vi "Dashboard Main.vi"() -> ()   [LabVIEW 2013]
uses:
  <vilib>/event_ctls.llb/eventvkey.ctl
  <vilib>/Rock Robotics/WPI/Dashboard/WPI_DashboardLogging Global.vi
  <vilib>/Utility/config.llb/Write Key (String).vi
  <vilib>/Utility/config.llb/Write Key (I32).vi
  <vilib>/Utility/config.llb/NI_LVConfig.lvlib
  <vilib>/vision/NI_Vision_Development_Module.lvlib
panel:
  out "Image Message":string="Timeout in Camera Communications"
  in  "Rec Mode":enum32{"Stop", "Record", "Playback"}(radio)
  in  "Dashboard Tab":T1(tab)=enum."Auto"
  out "SHOOT":bool
  in  "Camera Settings":T2={"Frame Rate"=7, "Compression"=0, "Size"=1} {"Frame Rate" scale=1.0..30.0; "Size" items=["640x480", "320x240", "160x120"]}
  out "MotorSliders R":cluster{"MotorSlide1":dbl, "MotorSlide2":dbl} {"MotorSlide2" scale=-1.0..1.0 scale format="%#_2e"; "MotorSlide1" scale=-1.0..1.0 scale format="%#_2e"}
  out "MotorChart R":cluster{"Numeric":dbl, "Numeric":dbl}(graph)
  out "MotorSliders L":T3 {"MotorSlide4 2" scale=0.0..14.0 scale format="%#_2e"; "MotorSlide2" scale=-1.0..1.0 scale format="%#_2e"; "MotorSlide1" scale=-1.0..1.0 scale format="%#_2e"}
  out "MotorChart L":T4(graph)
  out "JS1 Z":dbl(slide) scale=-1.0..1.0 scale format="%#_2e"
  out "Joystick 1":cluster{"X":dbl, "Y":dbl}[](graph)
  out "JS Buttons 1":T5
  out "JS2 Z":dbl(slide) scale=-1.0..1.0 scale format="%#_2e"
  out "Joystick 2":cluster{"X":dbl, "Y":dbl}[](graph)
  out "JS Buttons 2":T5
  out "Mode":T6(ring)=enum.""
  in  "DB Camera Config":bool
  out "fps":dbl format="%#.1g"
  out "Mbps":dbl format="%#.1g"
  out "Mbps 2":bool
  out "LED 1":bool
  out "Camera IP Address":string="0.0.0.11"
  in  "Bunches of Variables":T7={"Parameter 1"=1.0596, "Parameter 2"=-19.179, "Camera view angle"=33.7} {"Camera view angle" format="%#_13g"}
  out "Number of Particles":i32=1
  in  "Color Mode":u16(ring)=1 items=["RGB", "HSL", "HSV", "HSI"]
  out "Distance (in)":dbl
  in  "Filter ON":bool
  in  "Green or Saturation":cluster{i32, i32}(slide)={44, 255} scale=0.0..255.0
  in  "Blue or Luminance":cluster{i32, i32}(slide)={147, 255} scale=0.0..255.0
  in  "Red or Hue":cluster{i32, i32}(slide)={89, 148} scale=0.0..255.0
  in  "Combo Box":string(combo)="Custom"
  out "Tallest Area":dbl
  out "Widest Area":dbl
  out "Hot":bool
  in  "Test Slider":dbl(slide) scale=0.0..100.0 scale format="%#_3g"
  in  "On/Off":bool caption="Solenoid"
  in  "Test Name":u16(ring) items=["Select the test to run...", "Example Test", "-------------------------------", "List of tests is built in robot code.", "Replace with your own automated tests."]
  in  "Test Tree":string(tree)
  in  "Motor":cluster{"Value":dbl, "Enable":bool} {"Value" scale=-1.0..1.0 scale format="%#_3g"}
  out "Progress":T8 {"Test Progress" scale=0.0..100.0}
  in  "Rev/Fwd":cluster{"Forward":bool, "Reverse":bool}
  in  "Test Ring":u16(ring) items=["Auto", "Fixed indoor", "Fixed outdoor 1", "Fixed outdoor 2", "Fixed fluorescent 1", "Fixed fluorescent 2", "Hold current"]
  in  "Listbox":i32(listbox)
  out "Tree":string(tree)
  out "Camera Image":T9(plugin-control)
  # "Left"
  # "Front"
  # "Right"
  # "Battery"
  # "Customize by placing controls and indicators here and name to\nmatch Dashboard Variables on robot."
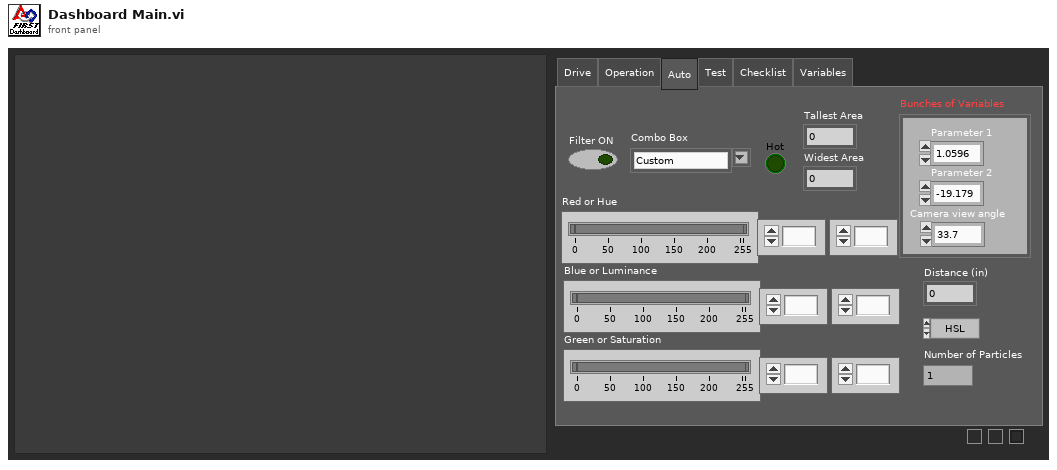
[diagram p1: front panel]
types:
  T1 = enum32{"Drive", "Operation", "Auto", "Test", "Checklist", "Variables"}
  T2 = cluster{"Frame Rate":i32, "Compression":i32, "Size":u16}
  T3 = cluster{"MotorSlide1":dbl, "MotorSlide2":dbl, "MotorSlide4 2":dbl}
  T4 = cluster{"Numeric":dbl, "Numeric":dbl, "Battery":sgl}
  T5 = cluster{bool, bool, bool, bool, bool, bool, bool, bool, bool, bool, bool, bool}
  T6 = enum8{"Tele-Op Disabled", "Tele-Op Enabled", "Auto Disabled", "Auto Enabled", "Test Disabled", "Test Enabled", ""}
  T7 = cluster{"Parameter 1":dbl, "Parameter 2":dbl, "Camera view angle":dbl}
  T8 = cluster{"Test Progress":u8, "Test Progress Text":string}
  T9 = typedef "IMAQ Image.ctl" = refnum<image>
  T10 = typedef "Image Type" = u32
  T11 = cluster{"Digital Inputs":bool[], "Digital Outputs":bool[]}
  T12 = cluster{"Competition mode":bool, "Robot Link":bool, "Autonomous":bool, "Enabled":bool, "E-Stop":bool, "Simulated":bool, "TestMode":bool, "Docked Window":bool}
  T13 = cluster{"Boolean Array[0]":bool, "Boolean Array[1]":bool, "Boolean Array[2]":bool, "Boolean Array[3]":bool, "Boolean Array[4]":bool, "Boolean Array[5]":bool, "Boolean Array[6]":bool, "Boolean Array[7]":bool, "Boolean Array[8]":bool, "Boolean Array[9]":bool, "Boolean Array[10]":bool, "Boolean Array[11]":bool}
  T14 = typedef "NI_LVConfig.lvlib/Config Data RefNum.ctl" = refnum<k1>
  T15 = typedef "eventvkey.ctl" = enum16{"ASCII", "Enter", "Return", "Shift", "Ctrl", "Alt", "Cmd", "Opt", "Caps", "NumLock", "Clear", "Break", "Up", "Down", "Left", "Right", "Insert", "Delete", "Home", "End", "PageUp", "PageDown", "Escape", "Help", "Pause", "ScrollLock", "F1", "F2", "F3", "F4", "F5", "F6", "F7", "F8", "F9", "F10", "F11", "F12", "F13", "F14", "F15", "F16", "F17", "F18", "F19", "F20", "F21", "F22", "F23", "F24", "Play", "VolumeUp", "VolumeDown", "Mute", "Two Byte Char"}
  T16 = cluster{"Image Size":bool, "Image Type":bool, "Pixel Value":bool, "ROI Information":bool, "Zoom Factor":bool}
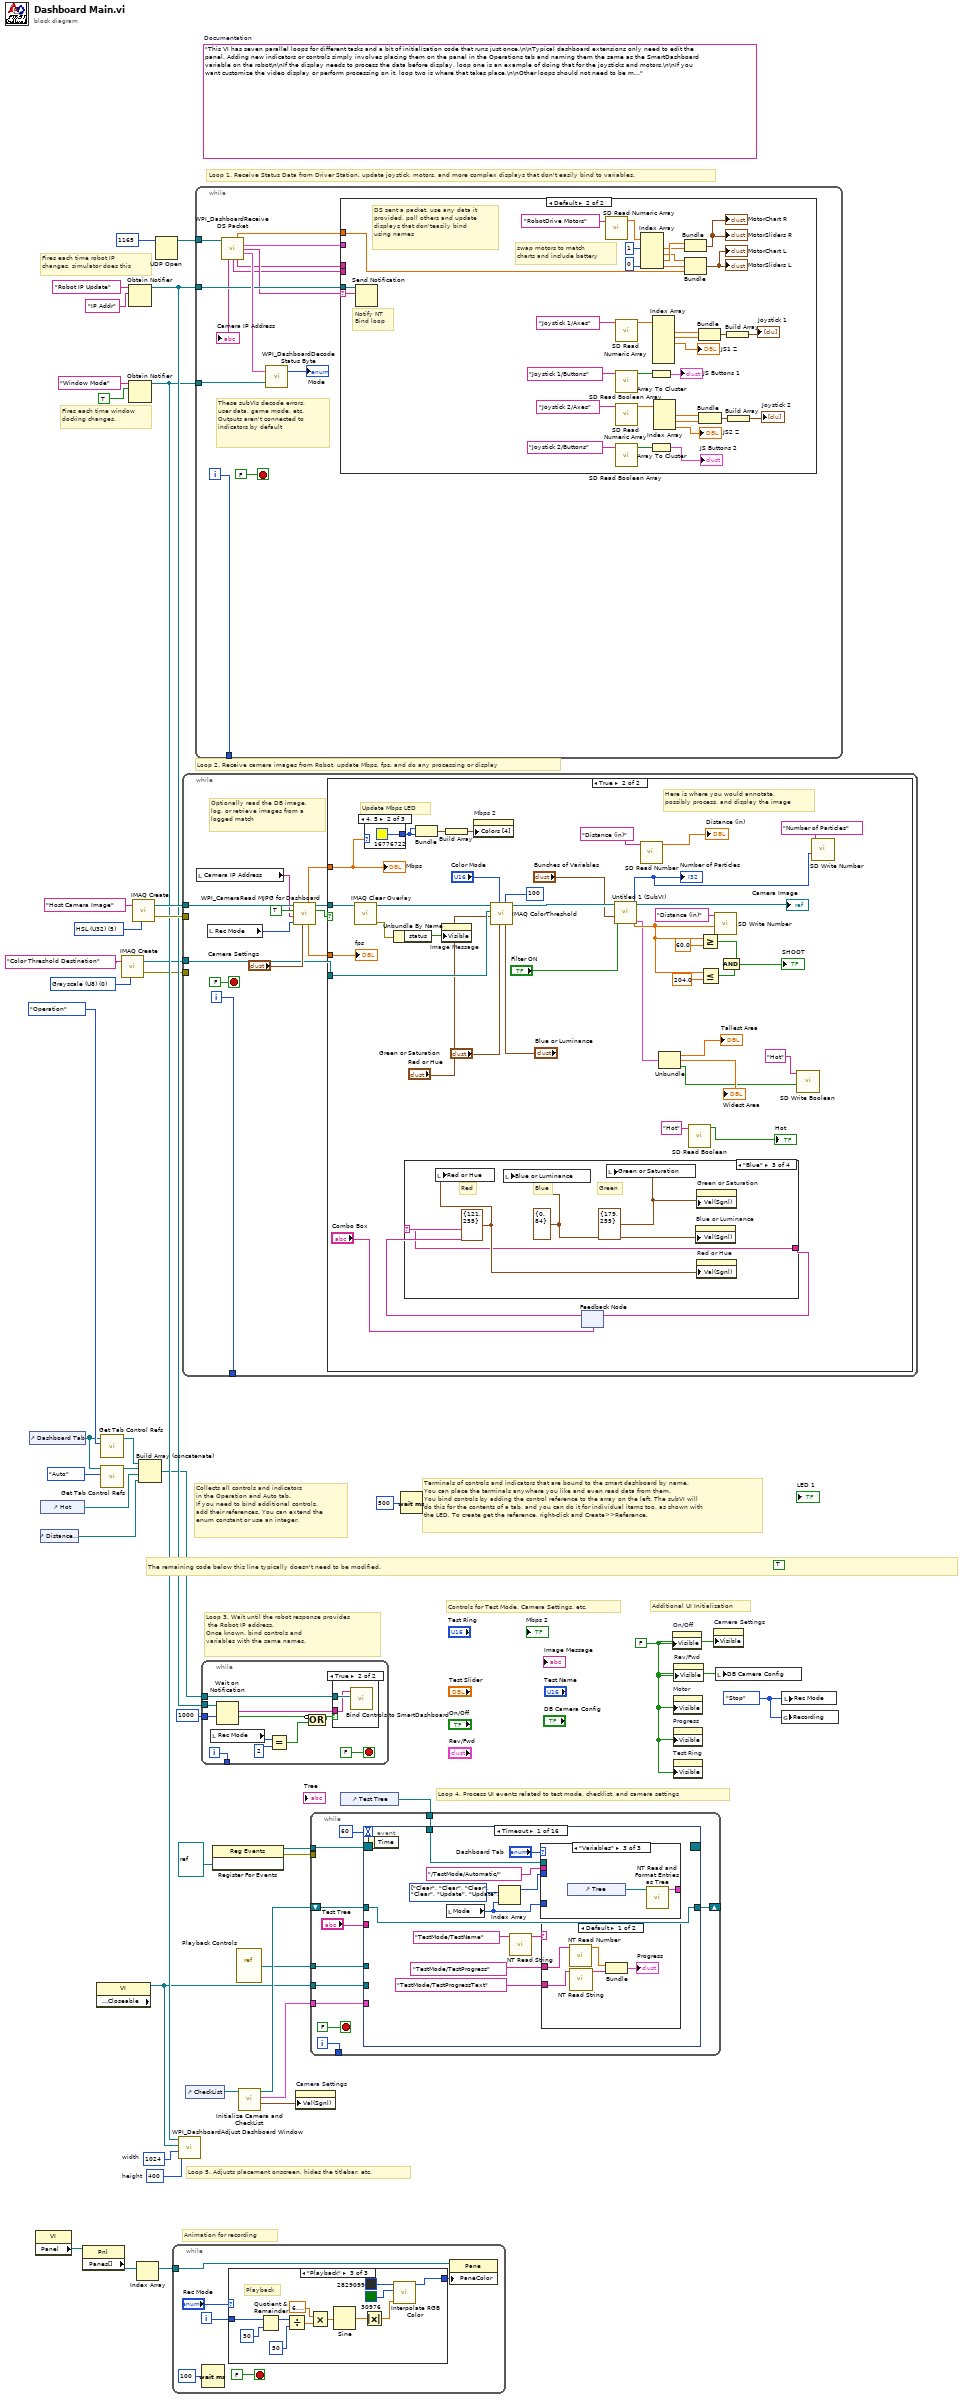
[diagram p0: block diagram]
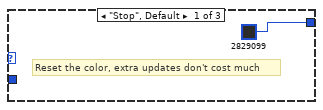
[diagram p2: hidden frame]
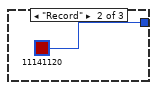
[diagram p3: hidden frame]
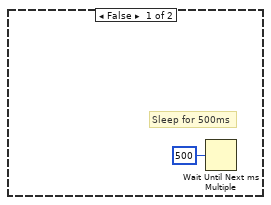
[diagram p5: hidden frame]
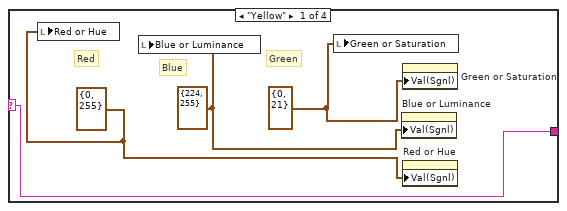
[diagram p6: hidden frame]
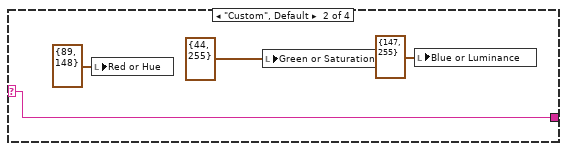
[diagram p7: hidden frame]
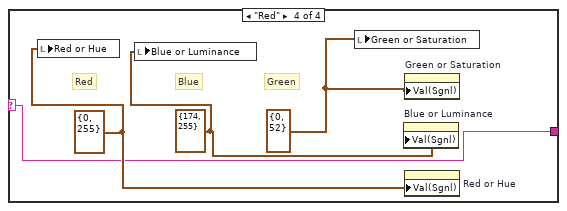
[diagram p8: hidden frame]
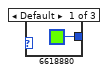
[diagram p9: hidden frame]
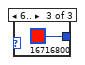
[diagram p10: hidden frame]
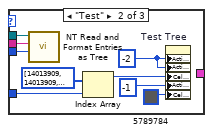
[diagram p12: hidden frame]
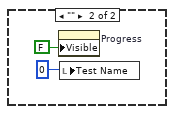
[diagram p13: hidden frame]
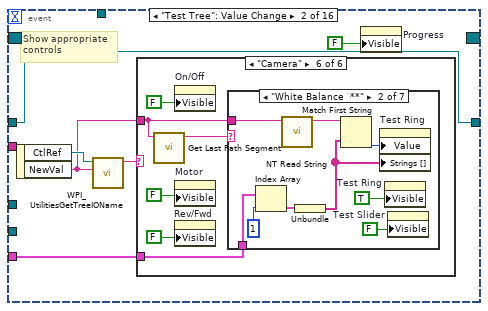
[diagram p14: hidden frame]
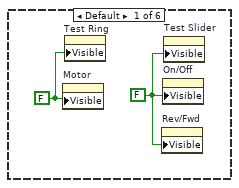
[diagram p15: hidden frame]
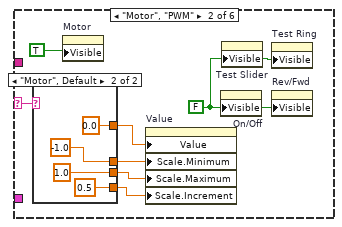
[diagram p16: hidden frame]
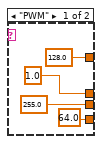
[diagram p17: hidden frame]
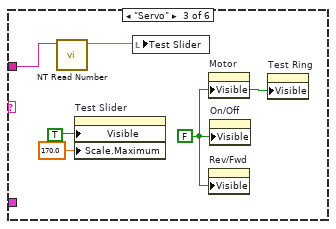
[diagram p18: hidden frame]
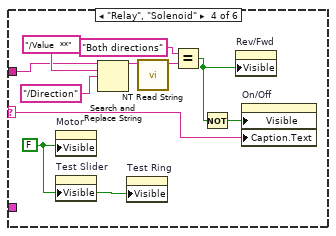
[diagram p19: hidden frame]
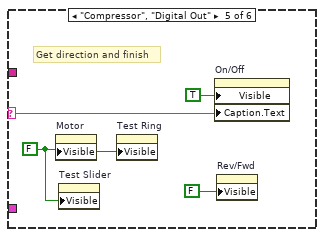
[diagram p20: hidden frame]
diagram:
  (unwired) TRUE
  w6 = T10 0 items=["Grayscale (U8)", "Grayscale (I16)", "Grayscale (SGL)", "Complex (CSG)", "RGB (U32)", "HSL (U32)", "RGB (U64)", "Grayscale (U16)"] ("Image Type")
  w14 = enum32{"Stop", "Record", "Playback"}."Stop" ("Rec Mode")
  w17 = 400  # height
  w18 = 1024  # width
  w31 = FALSE ("Visible")
  (unwired) "This VI has seven parallel loops for different tasks and a bit of initialization code that runs just once.\n\nTypical dashboard extensions only need to edit the panel. Adding new indicators or controls simply involves placing them on the panel in the Operations tab and naming them the same as the SmartDashboard variable on the robot\n\nIf the display needs to process the data before display, loop one is an example of doing that for the joysticks and motors.\n\nIf you want customize the video display or perform processing on it, loop two is where that takes place.\n\nOther loops should not need to be modified. They are pretty standard, and document the task they perform."  # Documentation
  w41 = T10 5 items=["Grayscale (U8)", "Grayscale (I16)", "Grayscale (SGL)", "Complex (CSG)", "RGB (U32)", "HSL (U32)", "RGB (U64)"] ("Image Type")
  # "Controls for Test Mode, Camera Settings, etc."
  # "Additional UI Initialization"
  # "Animation for recording"
  # "Fires each time robot IP\nchanges, simulator does this"
  # "Fires each time window\ndocking changes."
  # "Collects all controls and indicators\nin the Operation and Auto tab.\nIf you need to bind additional controls,\nadd their references. You can extend the\nenum constant or use an integer."
  # "The remaining code below this line typically doesn't need to be modified."
  # "Loop 4. Process UI events related to test mode, checklist, and camera settings"
  # "Terminals of controls and indicators that are bound to the smart dashboard by name.\nYou can place the terminals anywhere you like and even read data from them.\nYou bind controls by adding the control reference to the array on the left. The subVI will\ndo this for the contents of a tab, and you can do it for individual items too, as shown with\nthe LED. To create get the reference, right-click and Create>>Reference."
  # "Loop 3. Wait until the robot response provides\n the Robot IP address.\nOnce known, bind controls and\nvariables with the same names."
  # "Loop 5. Adjusts placement onscreen, hides the titlebar, etc."
  # "Loop 1. Receive Status Data from Driver Station, update joystick, motors, and more complex displays that don't easily bind to variables."
  # "Loop 2. Receive camera images from Robot, update Mbps, fps, and do any processing or display"
  n1 = control-ref of="Dashboard Tab"() -> (w12:refnum<vi>)
  n2 = property class="VI"() -> ("Panel"=w25:refnum<vi>)  [unwired: 2 in, 2 out]
  n3 = control-ref of="Hot"() -> (w7:refnum<vi>)
  n4 = control-ref of="Distance (in)"() -> (w2:refnum<vi>)
  n5 = property class="Pnl"(reference=w25) -> ("Panes[]"=w26:refnum<vi>[])  [unwired: 1 in, 2 out]
  n6 = property class="VI" props=["Front Panel.Closeable"]() -> (reference out=w13:refnum<vi>)  [unwired: 2 in, 2 out]
  n7 = call <vilib>:"Get Tab Control Refs.vi"("Page Index"=T1."Operation" ("Dashboard Tab"), "TabControl in"=w12) -> ("ControlsOnPage"=w10:refnum<vi>[])  [unwired: 9 in]
  n8 = call <vilib>:"Get Tab Control Refs.vi"("Page Index"=T1."Auto" ("Dashboard Tab"), "TabControl in"=w12) -> ("ControlsOnPage"=w11:refnum<vi>[])  [unwired: 9 in]
  n9 = call "IMAQ Create"("Image Name"="Color Threshold Destination", "Image Type"=w6) -> ("New Image"=w5:T9, "error out"=w4:errorcluster)  [unwired: 3 in]
  n10 = Obtain Notifier(name (unnamed)="Robot IP Update", notification data type="IP Addr" ("name (unnamed)")) -> (notifier out=w35:refnum<notifier>)  [unwired: 2 in, 2 out]
  n11 = Obtain Notifier(name (unnamed)="Window Mode", notification data type=TRUE) -> (notifier out=w16:refnum<notifier>)  [unwired: 2 in, 2 out]
  n12 = call "IMAQ Create"("Image Name"="Host Camera Image", "Image Type"=w41) -> ("New Image"=w39:T9, "error out"=w38:errorcluster)  [unwired: 2 in, 1 out]
  n13 = Index Array(array=w26) -> (element=w24:refnum<vi>)  [unwired: 1 in]
  n14 = Build Array (concatenate)(w10, w11, w7, w2) -> (w9:refnum<vi>[])
  n15 = UDP Open(11:u16 1165 ("port")) -> (port=w42:refnum<k16>)  [unwired: 2 in, 4 out]
  n16 = while {
    tunnel: w24 -> [w45]
    i -> [w48]
    stop <- FALSE stop-if-true
    n17 = Wait (ms)(milliseconds to wait=u32 100) -> ()  [unwired: 1 out]
    n18 = case shown="\"Playback\"" "Rec Mode" {
      tunnel: w48 -> [_ _ w63]
      tunnel: [u32 2829099 ("Base Color") u32 11141120 ("Target Color") w52] -> w44
      frame "Stop", Default {
        # "Reset the color, extra updates don't cost much"
      }
      frame "Record" {
      }
      frame "Playback" {
        # "Playback"
        n19 = Quotient & Remainder(x=w63, y=u32 50 ("milliseconds to wait")) -> (x-y*floor(x/y)=w59:u32)  [unwired: 1 out]
        n20 = Divide(x=w59, y=u32 50 ("milliseconds to wait")) -> (x/y=w56:dbl)
        n21 = Multiply(x=6.283185307179586, y=w56) -> (x*y=w61:dbl)
        n22 = Sine(x=w61) -> (sin(x)=w60:dbl)
        n23 = Absolute Value(x=w60) -> (abs(x)=w53:dbl)
        n24 = call "Interpolate RGB Color.vi"("Proportion"=w53, "Target Color"=u32 30976, "Base Color"=u32 2829099) -> ("Result Color"=w52:u32)  [unwired: 8 in]
      }
    }
    n25 = property class="Pane"(reference=w45, "PaneColor"=w44) -> ()  [unwired: 1 in, 2 out]
  }
  n26 = call <vilib>:"WPI_DashboardAdjust Dashboard Window.vi"("height"=w17, "width"=w18, "reference in"=w13, "Notifier in"=w16) -> ()  [unwired: 8 in]
  n27 = while {
    tunnel: w39 -> [w73]
    tunnel: w38 -> [_]
    tunnel: [w74] -> _
    tunnel: w5 -> [w66]
    tunnel: w4 -> [_]
    i -> [w74]
    stop <- FALSE stop-if-true
    # "Optionally read the DB image,\nlog, or retrieve images from a\nlogged match"
    n28 = local read "Camera IP Address"() -> (w64:string)
    n29 = local read "Rec Mode"() -> (w65:enum32{"Stop", "Record", "Playback"})
    n30 = call <vilib>:"WPI_CameraRead MJPG for Dashboard.vi"("Camera Settings"="Camera Settings", "Rec Mode"=w65, "Camera IP"=w64, "Enable"=TRUE, "Refnum in"=w73) -> ("Active"=w70:bool, "Refnum out"=w72:T9, "FPS"=w69:dbl, "Bandwidth (Mbps)"=w68:dbl)  [unwired: 3 in]
    n31 = case shown="True" w70 {
      tunnel: w72 -> [_ w111]
      tunnel: w68 -> [_ w110]
      tunnel: w69 -> [_ w109]
      tunnel: w66 -> [_ w106]
      frame False {
        # "Sleep for 500ms"
        n32 = Wait Until Next ms Multiple(millisecond multiple=u32 500) -> ()  [unwired: 1 out]
      }
      frame True {
        # "Here is where you would annotate,\npossibly process, and display the image"
        # "Update Mbps LED"
        n33 = call "IMAQ Clear Overlay"("Image"=w111) -> ("error out"=w115:errorcluster, "Image Out"=w105:T9)  [unwired: 2 in, 7 out]
        n34 = case shown="4, 5" w110 {
          tunnel: [u32 6618880 ("Color Box") u32 16776722 ("Color Box") u32 16716800 ("Color Box")] -> w112
          frame Default {
          }
          frame 4, 5 {
          }
          frame 6.. {
          }
        }
        n35 = Unbundle By Name(w115) -> ("status"=w116:bool)
        n36 = Bundle("Color Box"=w112, "Color Box"=w112) -> (w114:cluster{"Color Box":u32, "Color Box":u32})  [unwired: 1 out]
        n37 = property on="Image Message" class="Str"("Visible"=w116) -> ()  [unwired: 2 in, 2 out]
        n38 = Build Array(w114) -> (w113:cluster{"Color Box":u32, "Color Box":u32}[])
        n39 = property on="Mbps 2" class="Bool (strict)"("Colors [4]"=w113) -> ()  [unwired: 2 in, 2 out]
        n40 = call "IMAQ ColorThreshold"("Blue or Luma or Val or Inten Range"="Blue or Luminance", "Replace Value"=100, "Green or Sat Range"="Green or Saturation", "Color Mode"="Color Mode", "Red or Hue Range"="Red or Hue", "Image Dst"=w106, "Image Src"=w105) -> ("Image Dst Out"=w104:T9)  [unwired: 3 in, 1 out]
        n41 = feedback #1("Combo Box") -> (w84:string)
        n42 = case shown="\"Blue\"" w84 {
          selector: w84 -> [w117 w121 w125 w129]
          tunnel: [w117 w121 w125 w129] -> w85
          frame "Yellow" {
            w118 = cluster{"Lower value":i32, "Upper value":i32} {"Lower value"=0, "Upper value"=21} ("Red or Hue Range")
            w119 = cluster{"Lower value":i32, "Upper value":i32} {"Lower value"=224, "Upper value"=255} ("Red or Hue Range")
            w120 = cluster{"Lower value":i32, "Upper value":i32} {"Lower value"=0, "Upper value"=255} ("Red or Hue Range")
            # "Green"
            # "Blue"
            # "Red"
            n43 = local write "Red or Hue"(w120) -> ()
            n44 = local write "Blue or Luminance"(w119) -> ()
            n45 = local write "Green or Saturation"(w118) -> ()
            n46 = property on="Blue or Luminance" class="Slide (strict)"("Val(Sgnl)"=w119) -> ()  [unwired: 2 in, 2 out]
            n47 = property on="Green or Saturation" class="Slide (strict)"("Val(Sgnl)"=w118) -> ()  [unwired: 2 in, 2 out]
            n48 = property on="Red or Hue" class="Slide (strict)"("Val(Sgnl)"=w120) -> ()  [unwired: 2 in, 2 out]
          }
          frame "Custom", Default {
            n49 = local write "Red or Hue"(cluster{i32, i32} {89, 148} ("Red or Hue")) -> ()
            n50 = local write "Green or Saturation"(cluster{i32, i32} {44, 255} ("Green or Saturation")) -> ()
            n51 = local write "Blue or Luminance"(cluster{i32, i32} {147, 255} ("Blue or Luminance")) -> ()
          }
          frame "Blue" {
            w127 = cluster{"Lower value":i32, "Upper value":i32} {"Lower value"=179, "Upper value"=255} ("Red or Hue Range")
            w128 = cluster{"Lower value":i32, "Upper value":i32} {"Lower value"=0, "Upper value"=84} ("Red or Hue Range")
            w126 = cluster{"Lower value":i32, "Upper value":i32} {"Lower value"=121, "Upper value"=255} ("Red or Hue Range")
            # "Green"
            # "Blue"
            # "Red"
            n52 = local write "Red or Hue"(w126) -> ()
            n53 = local write "Blue or Luminance"(w128) -> ()
            n54 = local write "Green or Saturation"(w127) -> ()
            n55 = property on="Blue or Luminance" class="Slide (strict)"("Val(Sgnl)"=w128) -> ()  [unwired: 2 in, 2 out]
            n56 = property on="Green or Saturation" class="Slide (strict)"("Val(Sgnl)"=w127) -> ()  [unwired: 2 in, 2 out]
            n57 = property on="Red or Hue" class="Slide (strict)"("Val(Sgnl)"=w126) -> ()  [unwired: 2 in, 2 out]
          }
          frame "Red" {
            w131 = cluster{"Lower value":i32, "Upper value":i32} {"Lower value"=0, "Upper value"=52} ("Red or Hue Range")
            w132 = cluster{"Lower value":i32, "Upper value":i32} {"Lower value"=174, "Upper value"=255} ("Red or Hue Range")
            w130 = cluster{"Lower value":i32, "Upper value":i32} {"Lower value"=0, "Upper value"=255} ("Red or Hue Range")
            # "Green"
            # "Blue"
            # "Red"
            n58 = local write "Red or Hue"(w130) -> ()
            n59 = local write "Blue or Luminance"(w132) -> ()
            n60 = local write "Green or Saturation"(w131) -> ()
            n61 = property on="Blue or Luminance" class="Slide (strict)"("Val(Sgnl)"=w132) -> ()  [unwired: 2 in, 2 out]
            n62 = property on="Green or Saturation" class="Slide (strict)"("Val(Sgnl)"=w131) -> ()  [unwired: 2 in, 2 out]
            n63 = property on="Red or Hue" class="Slide (strict)"("Val(Sgnl)"=w130) -> ()  [unwired: 2 in, 2 out]
          }
        }
        n64 = feedback-in #1(w85) -> ()
        n65 = call "Untitled 1 (SubVI).vi"("Filter ON"="Filter ON", "Cluster"="Bunches of Variables", "Image Dst Out"=w104, "Refnum in"=w105) -> ("output cluster"=w88:cluster{dbl, dbl, bool}, "Distance (in)"=w94:dbl, "Number of Particles"=w77:i32, "Refnum out"=→"Camera Image":T9)  [unwired: 4 in]
        "Number of Particles" <- w77
        n66 = call <vilib>:"SD Read Number.vi"("Name"="Distance (in)") -> ("Numeric"=→"Distance (in)":dbl)  [unwired: 8 in, 2 out]
        n67 = Unbundle(w88) -> (→"Tallest Area":dbl, →"Widest Area":dbl, w82:bool)
        n68 = call <vilib>:"SD Read Boolean.vi"("Name"="Hot") -> ("Boolean"=→"Hot":bool)  [unwired: 8 in, 2 out]
        n69 = Greater Or Equal?(x=w94, y=60.0) -> (x >= y?=w102:bool)
        n70 = Less Or Equal?(x=w94, y=204.0) -> (x <= y?=w100:bool)
        n71 = call <vilib>:"SD Write Number.vi"("Numeric"=w94, "Name"="Distance (in)") -> ()  [unwired: 8 in, 2 out]
        n72 = And(x=w102, y=w100) -> (x .and. y?=→"SHOOT":bool)
        n73 = call <vilib>:"SD Write Boolean.vi"("Boolean"=w82, "Name"="Hot") -> ()  [unwired: 8 in, 2 out]
        n74 = call <vilib>:"SD Write Number.vi"("Numeric"=w77, "Name"="Number of Particles") -> ()  [unwired: 8 in, 2 out]
        "Mbps" <- w110
        "fps" <- w109
      }
    }
  }
  n75 = control-ref of="CheckList"() -> (w15:refnum<vi>)
  n76 = while {
    tunnel: w42 -> [w146]
    tunnel: w35 -> [w142]
    tunnel: w16 -> [w145]
    tunnel: [w143] -> _
    i -> [w143]
    stop <- FALSE stop-if-true
    # "These subVIs decode errors, user data, game mode, etc.\nOutputs aren't connected to indicators by default"
    n77 = call <vilib>:"WPI_DashboardReceive DS Packet.vi"("Recv Socket"=w146) -> ("Battery"=w137:sgl, "Driver Station"=w138:T11, "Robot IP Address"=w141:string, "Status"=w147:T12, "Camera IP Address"=→"Camera IP Address":string, "Low Priority User Data"=w140:string, "High Priority User Data"=w139:string)  [unwired: 1 in, 7 out]
    n78 = call <vilib>:"WPI_DashboardDecode Status Byte.vi"("Window Mode Notifier"=w145, "Status"=w147) -> ("Mode"=→"Mode":T6)  [unwired: 1 out]
    n79 = case shown="Default" w141 {
      selector: w141 -> [_ w159]
      tunnel: w142 -> [_ w160]
      tunnel: w140 -> [_ _]
      tunnel: w139 -> [_ _]
      tunnel: w138 -> [_ _]
      tunnel: w137 -> [_ w158]
      frame "0.0.0.0" {
        # "DS not sending packets, or no robot exists yet.\nDon't poll the variables"
      }
      frame Default {
        # "Notify NT\nBind loop"
        # "DS sent a packet. use any data it\nprovided, poll others and update\ndisplays that don'teasily bind\nusing names"
        # "swap motors to match\ncharts and include battery"
        n80 = Send Notification(notification=w159, notifier=w160) -> ()  [unwired: 1 in, 2 out]
        n81 = call <vilib>:"SD Read Numeric Array.vi"("Name"="RobotDrive Motors") -> ("Numeric Array"=w157:dbl[])  [unwired: 8 in, 2 out]
        n82 = call <vilib>:"SD Read Numeric Array.vi"("Name"="Joystick 1/Axes") -> ("Numeric Array"=w176:dbl[])  [unwired: 8 in, 2 out]
        n83 = call <vilib>:"SD Read Boolean Array.vi"("Name"="Joystick 1/Buttons") -> ("Boolean Array"=w178:bool[])  [unwired: 8 in, 2 out]
        n84 = call <vilib>:"SD Read Numeric Array.vi"("Name"="Joystick 2/Axes") -> ("Numeric Array"=w170:dbl[])  [unwired: 8 in, 2 out]
        n85 = call <vilib>:"SD Read Boolean Array.vi"("Name"="Joystick 2/Buttons") -> ("Boolean Array"=w169:bool[])  [unwired: 8 in, 2 out]
        n86 = Index Array(array=w157, index #1=1, index #4=0) -> (element #1=w153:dbl, element #2=w152:dbl, element #3=w154:dbl, element #4=w149:dbl)  [unwired: 2 in]
        n87 = Array To Cluster(array=w178) -> (cluster=→"JS Buttons 1":T13)
        n88 = Array To Cluster(array=w169) -> (cluster=→"JS Buttons 2":T13)
        n89 = Index Array(array=w176) -> (element #1=w173:dbl, element #2=w174:dbl, element #3=→"JS1 Z":dbl)  [unwired: 6 in, 3 out]
        n90 = Index Array(array=w170) -> (element #1=w165:dbl, element #2=w164:dbl, element #3=→"JS2 Z":dbl)  [unwired: 3 in]
        n91 = Bundle("Numeric"=w154, "Numeric"=w153) -> (→"MotorChart R" →"MotorSliders R":cluster{"Numeric":dbl, "Numeric":dbl})  [unwired: 1 in]
        n92 = Bundle("Numeric"=w152, "Numeric"=w149, "Battery"=w158) -> (→"MotorChart L" →"MotorSliders L":T4)  [unwired: 1 in]
        n93 = Bundle("Numeric"=w173, "Numeric"=w174) -> (w172:cluster{"Numeric":dbl, "Numeric":dbl})  [unwired: 1 in]
        n94 = Bundle("Numeric"=w165, "Numeric"=w164) -> (w166:cluster{"Numeric":dbl, "Numeric":dbl})  [unwired: 1 in]
        n95 = Build Array(w172) -> (→"Joystick 1":cluster{"Numeric":dbl, "Numeric":dbl}[])
        n96 = Build Array(w166) -> (→"Joystick 2":cluster{"Numeric":dbl, "Numeric":dbl}[])
      }
    }
  }
  n97 = while {
    tunnel: w9 -> [w192]
    tunnel: w35 -> [w190]
    tunnel: [w188] -> _
    tunnel: u32 1000 ("milliseconds to wait") -> [w187]
    i -> [w188]
    stop <- FALSE stop-if-true
    n98 = local read "Rec Mode"() -> (w183:enum32{"Stop", "Record", "Playback"})
    n99 = Wait on Notification(notifier=w190, timeout in ms (-1)=w187) -> (notification=w189:string, timed out?=w185:bool)  [unwired: 2 in, 2 out]
    n100 = Equal?(x=w183, y=u16 2 ("Rec Mode")) -> (x = y?=w184:bool)
    n101 = Compound Arithmetic op=OR(invert w185, w184) -> (w186:bool)
    n102 = case shown="True" w186 {
      tunnel: w192 -> [_ w194]
      tunnel: w189 -> [_ w193]
      frame False {
      }
      frame True {
        n103 = call <vilib>:"Bind Controls to SmartDashboard.vi"("Bound Control Refs"=w194, "Server IP Address"=w193) -> ()  [unwired: 10 in]
      }
    }
  }
  n104 = register-events(refnum<vi> refnum) -> (reference out=w22:refnum<event-registration>, error out=w21:errorcluster)  [unwired: 2 in]
  n105 = vi-ref "Playback Controls.vi"() -> (w23:refnum<vi>)
  n106 = call "Initialize Camera and CheckList.vi"("ListBox in"=w15) -> ("Cluster"=w29:cluster{"value":i32, "value":i32, "index":i32}, "Array"=w30:cluster{string[]}[], "File Refnum"=w28:T14)  [unwired: 8 in]
  n107 = property on="Camera Settings" class="Clust (strict)"("Val(Sgnl)"=w29) -> ()  [unwired: 2 in, 2 out]
  n108 = control-ref of="Test Tree"() -> (w27:refnum<vi>)
  n109 = while {
    tunnel: w30 -> [w202]
    shift-right: [w201] -> _
    shift-left: w28 -> [w200]
    tunnel: [w199] -> _
    tunnel: w27 -> [w198]
    tunnel: w23 -> [w197]
    tunnel: w22 -> [w196]
    tunnel: w21 -> [_]
    tunnel: w13 -> [w195]
    i -> [w199]
    stop <- FALSE stop-if-true
    n110 = event shown="[0] Timeout" {
      selector: w196 -> [_ _ _ _ _ _ _ _ _ _ _ _ _ _ _ _]
      dyn-events: [_ _ _ _ _ _ _ _ _ _ _ _ _ w440 _ _] -> _
      timeout: u32 60 ("milliseconds to wait") -> [_ _ _ _ _ _ _ _ _ _ _ _ _ _ _ _]
      tunnel: w198 -> [w212 _ _ _ _ _ _ _ _ _ _ _ _ _ _ _]
      tunnel: "Test Tree" -> [_ _ _ _ _ _ _ _ w409 w417 w419 w423 w431 _ _ _]
      tunnel: w202 -> [_ w236 _ _ _ _ w373 w403 _ _ _ _ _ _ _ _]
      tunnel: [w206 w235 w334 w339 w347 w359 w372 w396 w408 w415 w418 w422 w430 w442 w456 w457] -> w201
      tunnel: w200 -> [w206 w235 w334 w339 w347 w359 w371 w396 w408 w415 w418 w422 w430 w442 w456 w457]
      tunnel: w197 -> [_ _ _ _ _ _ _ _ _ _ _ _ _ w443 _ w460]
      tunnel: w195 -> [_ _ _ _ _ _ _ _ _ _ _ _ _ w438 _ _]
      event Timeout {
        w211 = enum16{"Update", "Clear"}[] [enum."Clear", enum."Clear", enum."Clear", enum."Clear", enum."Update", enum."Update", enum."Clear"] items=["Update", "Clear"]
        n111 = event-data() -> ()  [unwired: 1 in, 1 out]
        n112 = local read "Mode"() -> (w209:T6)
        n113 = Index Array(array=w211, index=w209) -> (element=w210:enum16{"Update", "Clear"})
        n114 = call <vilib>:"NT Read String.vi"("Name"="TestMode/TestName") -> ("String"=w215:string)  [unwired: 9 in, 1 out]
        n115 = case shown="\"Variables\"" "Dashboard Tab" {
          tunnel: w212 -> [_ w225 _]
          tunnel: "/TestMode/Automatic/" ("Name Pattern") -> [_ w224 _]
          tunnel: w210 -> [_ w223 _]
          tunnel: w209 -> [_ w221 _]
          tunnel: [_ _ w227] -> _
          frame "Operation", Default {
          }
          frame "Test" {
            w220 = -2 ("Active Item:Row Number")
            n116 = call <vilib>:"NT Read and Format Entries as Tree.vi"("Operation"=w223, "Name Pattern"=w224, "Tree Refnum"=w225) -> ()  [unwired: 7 in, 2 out]
            n117 = Index Array(array=u32[] [14013909, 14013909, 14013909, 14013909, 14013909, 16777215, 14013909], index=w221) -> (element=w219:u32)
            n118 = property on="Test Tree" class="Tree (strict)"("Active Item Row Number"=w220, "ActiveColNum"=w220, "CellBG"=w219, "Active Item Row Number"=-1 ("Active Item:Row Number"), "CellBG"=u32 5789784 ("Color Box")) -> ()  [unwired: 2 in, 2 out]
          }
          frame "Variables" {
            n119 = control-ref of="Tree"() -> (w226:refnum<vi>)
            n120 = call <vilib>:"NT Read and Format Entries as Tree.vi"("Tree Refnum"=w226) -> ("Formatted Strings"=w227:cluster{"Name":string, "Value":string}[])  [unwired: 9 in, 1 out]
          }
        }
        n121 = case shown="Default" w215 {
          tunnel: "TestMode/TestProgress" ("Name") -> [w229 _]
          tunnel: "TestMode/TestProgressText" ("Name") -> [w228 _]
          frame Default {
            n122 = call <vilib>:"NT Read Number.vi"("Name"=w229) -> ("Numeric"=w230:dbl)  [unwired: 9 in, 1 out]
            n123 = call <vilib>:"NT Read String.vi"("Name"=w228) -> ("String"=w231:string)  [unwired: 9 in, 1 out]
            n124 = Bundle("Numeric"=w230, "String"=w231) -> (→"Progress":cluster{"Numeric":dbl, "String":string})  [unwired: 1 in]
          }
          frame "" {
            n125 = property on="Progress" class="Clust (strict)"("Visible"=FALSE) -> ()  [unwired: 2 in, 2 out]
            n126 = local write "Test Name"(u16 0) -> ()
          }
        }
      }
      event "Test Tree": Value Change {
        # "Show appropriate\ncontrols"
        n127 = event-data() -> ("CtlRef"=w239:refnum<vi>, "NewVal"=w237:string)  [unwired: 1 in]
        n128 = call <vilib>:"WPI_UtilitiesGetTreeIOName.vi"("NewVal"=w237, "TreeControl in"=w239) -> ("I/O Name"=w240:string)  [unwired: 9 in]
        n129 = case shown="\"Camera\"" w240 {
          selector: w240 -> [_ w247 _ w265 w274 _]
          tunnel: w237 -> [_ _ w262 w264 _ w281]
          tunnel: w236 -> [_ _ _ _ _ w280]
          frame Default {
            w242 = FALSE ("Visible")
            w241 = FALSE ("Visible")
            n130 = property on="Motor" class="Clust (strict)"("Visible"=w241) -> ()  [unwired: 2 in, 2 out]
            n131 = property on="Test Ring" class="Ring (strict)"("Visible"=w241) -> ()  [unwired: 2 in, 2 out]
            n132 = property on="Rev/Fwd" class="Clust (strict)"("Visible"=w242) -> ()  [unwired: 2 in, 2 out]
            n133 = property on="On/Off" class="Bool (strict)"("Visible"=w242) -> ()  [unwired: 2 in, 2 out]
            n134 = property on="Test Slider" class="Slide (strict)"("Visible"=w242) -> ()  [unwired: 2 in, 2 out]
          }
          frame "Motor", "PWM" {
            w248 = FALSE ("Visible")
            n135 = case shown="\"Motor\", Default" w247 {
              tunnel: [1.0 ("Value") -1.0 ("Value")] -> w246
              tunnel: [255.0 ("Value") 1.0 ("Value")] -> w245
              tunnel: [128.0 ("Value") 0.0 ("Value")] -> w244
              tunnel: [64.0 ("Value") 0.5 ("Value")] -> w243
              frame "PWM" {
              }
              frame "Motor", Default {
              }
            }
            n136 = property on="Motor" class="Clust (strict)"("Visible"=TRUE) -> ()  [unwired: 2 in, 2 out]
            n137 = property on="Value" class="Slide (strict)"("Value"=w244, "Scale.Minimum"=w246, "Scale.Maximum"=w245, "Scale.Increment"=w243) -> ()  [unwired: 2 in, 2 out]
            n138 = property on="On/Off" class="Bool (strict)"("Visible"=w248) -> ()  [unwired: 2 in, 2 out]
            n139 = property on="Test Slider" class="Slide (strict)"("Visible"=w248) -> ()  [unwired: 2 in, 2 out]
            n140 = property on="Test Ring" class="Ring (strict)"("Visible"=w248) -> ()  [unwired: 2 in, 2 out]
            n141 = property on="Rev/Fwd" class="Clust (strict)"("Visible"=w248) -> ()  [unwired: 2 in, 2 out]
          }
          frame "Servo" {
            w260 = FALSE ("Visible")
            n142 = call <vilib>:"NT Read Number.vi"("Name"=w262) -> ("Numeric"=w261:dbl)  [unwired: 9 in, 1 out]
            n143 = property on="Test Slider" class="Slide (strict)"("Visible"=TRUE, "Scale.Maximum"=170.0 ("Scale.Range:Maximum")) -> ()  [unwired: 2 in, 2 out]
            n144 = local write "Test Slider"(w261) -> ()
            n145 = property on="Motor" class="Clust (strict)"("Visible"=w260) -> ()  [unwired: 2 in, 2 out]
            n146 = property on="Rev/Fwd" class="Clust (strict)"("Visible"=w260) -> ()  [unwired: 2 in, 2 out]
            n147 = property on="On/Off" class="Bool (strict)"("Visible"=w260) -> ()  [unwired: 2 in, 2 out]
            n148 = property on="Test Ring" class="Ring (strict)"("Visible"=w260) -> ()  [unwired: 2 in, 2 out]
          }
          frame "Relay", "Solenoid" {
            w263 = FALSE ("Visible")
            n149 = property on="Motor" class="Clust (strict)"("Visible"=w263) -> ()  [unwired: 2 in, 2 out]
            n150 = property on="Test Slider" class="Slide (strict)"("Visible"=w263) -> ()  [unwired: 2 in, 2 out]
            n151 = Search and Replace String(input string=w264, search string="/Value  **", replace string="/Direction") -> (result string=w270:string)  [unwired: 5 in, 3 out]
            n152 = property on="Test Ring" class="Ring (strict)"("Visible"=w263) -> ()  [unwired: 2 in, 2 out]
            n153 = call <vilib>:"NT Read String.vi"("Name"=w270) -> ("String"=w268:string)  [unwired: 9 in, 1 out]
            n154 = Equal?(x="Both directions", y=w268) -> (x = y?=w266:bool)
            n155 = Not(x=w266) -> (.not. x?=w267:bool)
            n156 = property on="Rev/Fwd" class="Clust (strict)"("Visible"=w266) -> ()  [unwired: 2 in, 2 out]
            n157 = property on="On/Off" class="Bool (strict)"("Visible"=w267, "Caption.Text"=w265) -> ()  [unwired: 2 in, 2 out]
          }
          frame "Compressor", "Digital Out" {
            w273 = FALSE ("Visible")
            # "Get direction and finish"
            n158 = property on="Motor" class="Clust (strict)"("Visible"=w273) -> ()  [unwired: 2 in, 2 out]
            n159 = property on="Test Slider" class="Slide (strict)"("Visible"=w273) -> ()  [unwired: 2 in, 2 out]
            n160 = property on="Test Ring" class="Ring (strict)"("Visible"=w273) -> ()  [unwired: 2 in, 2 out]
            n161 = property on="On/Off" class="Bool (strict)"("Visible"=TRUE, "Caption.Text"=w274) -> ()  [unwired: 2 in, 2 out]
            n162 = property on="Rev/Fwd" class="Clust (strict)"("Visible"=FALSE) -> ()  [unwired: 2 in, 2 out]
          }
          frame "Camera" {
            n163 = call <vilib>:"Get Last Path Segment.vi"("String in"=w281) -> ("String out"=w282:string)  [unwired: 10 in]
            n164 = property on="On/Off" class="Bool (strict)"("Visible"=FALSE) -> ()  [unwired: 2 in, 2 out]
            n165 = property on="Motor" class="Clust (strict)"("Visible"=FALSE) -> ()  [unwired: 2 in, 2 out]
            n166 = property on="Rev/Fwd" class="Clust (strict)"("Visible"=FALSE) -> ()  [unwired: 2 in, 2 out]
            n167 = case shown="\"White Balance  **\"" w282 {
              tunnel: w281 -> [w288 w297 w306 w315 w324 _ w330]
              tunnel: w280 -> [w286 w294 w303 w312 w321 _ _]
              frame "Size  **" {
                n168 = Index Array(array=w286) -> (element=w285:cluster{string[]})  [unwired: 1 in]
                n169 = call <vilib>:"NT Read String.vi"("Name"=w288) -> ("String"=w287:string)  [unwired: 9 in, 1 out]
                n170 = Unbundle(w285) -> (w283:string[])
                n171 = Match First String(2:w283, 3:w287) -> (0:w284:i32)  [unwired: 1 out]
                n172 = property on="Test Ring" class="Ring (strict)"("Value"=w284, "Strings []"=w283) -> ()  [unwired: 2 in, 2 out]
                n173 = property on="Test Ring" class="Ring (strict)"("Visible"=TRUE) -> ()  [unwired: 2 in, 2 out]
                n174 = property on="Test Slider" class="Slide (strict)"("Visible"=FALSE) -> ()  [unwired: 2 in, 2 out]
              }
              frame "White Balance  **" {
                n175 = Index Array(array=w294, index=1) -> (element=w295:cluster{string[]})
                n176 = call <vilib>:"NT Read String.vi"("Name"=w297) -> ("String"=w296:string)  [unwired: 9 in, 1 out]
                n177 = Unbundle(w295) -> (w292:string[])
                n178 = Match First String(2:w292, 3:w296) -> (0:w291:i32)  [unwired: 1 out]
                n179 = property on="Test Ring" class="Ring (strict)"("Value"=w291, "Strings []"=w292) -> ()  [unwired: 2 in, 2 out]
                n180 = property on="Test Ring" class="Ring (strict)"("Visible"=TRUE) -> ()  [unwired: 2 in, 2 out]
                n181 = property on="Test Slider" class="Slide (strict)"("Visible"=FALSE) -> ()  [unwired: 2 in, 2 out]
              }
              frame "Exposure  **" {
                n182 = Index Array(array=w303, index=2) -> (element=w304:cluster{string[]})
                n183 = call <vilib>:"NT Read String.vi"("Name"=w306) -> ("String"=w305:string)  [unwired: 9 in, 1 out]
                n184 = Unbundle(w304) -> (w300:string[])
                n185 = Match First String(2:w300, 3:w305) -> (0:w301:i32)  [unwired: 1 out]
                n186 = property on="Test Ring" class="Ring (strict)"("Value"=w301, "Strings []"=w300) -> ()  [unwired: 2 in, 2 out]
                n187 = property on="Test Ring" class="Ring (strict)"("Visible"=TRUE) -> ()  [unwired: 2 in, 2 out]
                n188 = property on="Test Slider" class="Slide (strict)"("Visible"=FALSE) -> ()  [unwired: 2 in, 2 out]
              }
              frame "Exposure Priority  **" {
                n189 = Index Array(array=w312, index=3) -> (element=w313:cluster{string[]})
                n190 = call <vilib>:"NT Read String.vi"("Name"=w315) -> ("String"=w314:string)  [unwired: 9 in, 1 out]
                n191 = Unbundle(w313) -> (w309:string[])
                n192 = Match First String(2:w309, 3:w314) -> (0:w310:i32)  [unwired: 1 out]
                n193 = property on="Test Ring" class="Ring (strict)"("Value"=w310, "Strings []"=w309) -> ()  [unwired: 2 in, 2 out]
                n194 = property on="Test Ring" class="Ring (strict)"("Visible"=TRUE) -> ()  [unwired: 2 in, 2 out]
                n195 = property on="Test Slider" class="Slide (strict)"("Visible"=FALSE) -> ()  [unwired: 2 in, 2 out]
              }
              frame "Color Enable  **" {
                n196 = Index Array(array=w321, index=4) -> (element=w322:cluster{string[]})
                n197 = call <vilib>:"NT Read String.vi"("Name"=w324) -> ("String"=w323:string)  [unwired: 9 in, 1 out]
                n198 = Unbundle(w322) -> (w318:string[])
                n199 = Match First String(2:w318, 3:w323) -> (0:w319:i32)  [unwired: 1 out]
                n200 = property on="Test Ring" class="Ring (strict)"("Value"=w319, "Strings []"=w318) -> ()  [unwired: 2 in, 2 out]
                n201 = property on="Test Ring" class="Ring (strict)"("Visible"=TRUE) -> ()  [unwired: 2 in, 2 out]
                n202 = property on="Test Slider" class="Slide (strict)"("Visible"=FALSE) -> ()  [unwired: 2 in, 2 out]
              }
              frame Default {
                n203 = property on="Test Ring" class="Ring (strict)"("Visible"=FALSE) -> ()  [unwired: 2 in, 2 out]
                n204 = property on="Test Slider" class="Slide (strict)"("Visible"=FALSE) -> ()  [unwired: 2 in, 2 out]
              }
              frame "Brightness  **", "Color Level  **", "Compression  **", "FPS  **", "Sharpness  **" {
                n205 = call <vilib>:"NT Read Number.vi"("Name"=w330) -> ("Numeric"=w329:dbl)  [unwired: 9 in, 1 out]
                n206 = local write "Test Slider"(w329) -> ()
                n207 = property on="Test Slider" class="Slide (strict)"("Visible"=TRUE, "Scale.Maximum"=100.0 ("Scale.Range:Maximum")) -> ()  [unwired: 2 in, 2 out]
                n208 = property on="Test Ring" class="Ring (strict)"("Visible"=FALSE) -> ()  [unwired: 2 in, 2 out]
              }
            }
          }
        }
        n209 = property on="Progress" class="Clust (strict)"("Visible"=FALSE) -> ()  [unwired: 2 in, 2 out]
      }
      event "Test Name": Mouse Enter {
        # "Populate the ring with the list of tests"
        n210 = event-data() -> ()  [unwired: 1 in, 1 out]
        n211 = call <vilib>:"NT Read String Array.vi"("Name"="TestMode/TestList") -> ("String Array"=w338:string[])  [unwired: 9 in, 1 out]
        n212 = Build Array (concatenate)("Select the test to run...", w338) -> (w337:string[])
        n213 = property on="Test Name" class="Ring (strict)"("Strings []"=w337) -> ()  [unwired: 2 in, 2 out]
      }
      event "Test Name": Value Change {
        w340 = FALSE ("Visible")
        # "Tell the robot the test name to run"
        n214 = event-data() -> ("NewVal"=w344:u16)  [unwired: 1 in]
        n215 = property on="Test Name" class="Ring (strict)"() -> ("Strings []"=w345:string[])  [unwired: 2 in, 2 out]
        n216 = local write "Progress"(T8 {"Test Progress"=0, "Test Progress Text"=""} ("Progress")) -> ()
        n217 = Index Array(array=w345, index=w344) -> (element=w343:string)
        n218 = call <vilib>:"NT Write String.vi"("String"=w343, "Name"="TestMode/TestName") -> ()  [unwired: 9 in, 1 out]
        n219 = property on="Progress" class="Clust (strict)"("Visible"=TRUE) -> ()  [unwired: 2 in, 2 out]
        n220 = property on="Motor" class="Clust (strict)"("Visible"=w340) -> ()  [unwired: 2 in, 2 out]
        n221 = property on="Test Slider" class="Slide (strict)"("Visible"=w340) -> ()  [unwired: 2 in, 2 out]
        n222 = property on="On/Off" class="Bool (strict)"("Visible"=w340) -> ()  [unwired: 2 in, 2 out]
        n223 = property on="Rev/Fwd" class="Clust (strict)"("Visible"=w340) -> ()  [unwired: 2 in, 2 out]
        n224 = property on="Test Ring" class="Ring (strict)"("Visible"=w340) -> ()  [unwired: 2 in, 2 out]
      }
      event "Listbox": Double Click {
        n225 = event-data() -> ("PlatMods.Shift"=w348:bool, "Row"=w350:i32)  [unwired: 1 in]
        n226 = case shown="True" w348 {
          tunnel: w350 -> [w354 _]
          tunnel: 1 -> [w353 _]
          frame False {
            n227 = property on="Listbox" class="LstBox (strict)"() -> ("Item Symbols"=w352:i32[])  [unwired: 2 in, 2 out]
            n228 = Replace Array Subset(array=w352, new element=w353, index=w354) -> (w351:i32[])
            n229 = property on="Listbox" class="LstBox (strict)"("Item Symbols"=w351) -> ()  [unwired: 2 in, 2 out]
          }
          frame True {
            w355 = 0 ("Top Row")
            n230 = property on="Listbox" class="LstBox (strict)"() -> ("Number of Rows"=w357:u32)  [unwired: 2 in, 2 out]
            n231 = Initialize Array(0, w357) -> (w356:i32[])
            n232 = property on="Listbox" class="LstBox (strict)"("Top Row"=w355, "Value"=w355, "Item Symbols"=w356) -> ()  [unwired: 2 in, 2 out]
          }
        }
      }
      event "Listbox": Key Down {
        n233 = event-data() -> ("VKey"=w361:T15)  [unwired: 1 in]
        n234 = case shown="\"Left\", \"Right\"" w361 {
          selector: w361 -> [w366 _]
          tunnel: eventvkey."Left" ("VKey") -> [w364 _]
          frame "Left", "Right" {
            n235 = Equal?(x=w364, y=w366) -> (x = y?=w365:bool)
            n236 = Select(t=0, s=w365, f=1) -> (s? t:f=w367:i32)
            n237 = property on="Listbox" class="LstBox (strict)"() -> ("Item Symbols"=w370:i32[])  [unwired: 2 in, 2 out]
            n238 = Replace Array Subset(array=w370, new element=w367, index="Listbox") -> (w369:i32[])
            n239 = property on="Listbox" class="LstBox (strict)"("Item Symbols"=w369) -> ()  [unwired: 2 in, 2 out]
          }
          frame Default {
          }
        }
      }
      event "DB Camera Config": Value Change {
        n240 = event-data() -> ("NewVal"=w374:bool)  [unwired: 1 in]
        n241 = case shown="False" w374 {
          tunnel: w373 -> [w383 _]
          tunnel: [w376 w394] -> w372
          tunnel: w371 -> [w375 w394]
          frame False {
            w390 = "Camera"
            w393 = FALSE ("Visible")
            n242 = local read "Camera Settings"() -> (w382:T2)
            n243 = Index Array(array=w383) -> (element=w386:cluster{string[]})  [unwired: 1 in]
            n244 = Unbundle(w382) -> ("Frame Rate"=w381:i32, "Compression"=w380:i32, "Size"=w384:u16)
            n245 = Unbundle(w386) -> (w385:string[])
            n246 = Index Array(array=w385, index=w384) -> (element=w379:string)
            n247 = call-poly <vilib>:"Write Key.vi"("section"=w390, "value"=w379, "key"="Size", "refnum"=w375) -> ("refnum out"=w392:T14)  [unwired: 2 in, 5 out]
            n248 = call-poly <vilib>:"Write Key.vi"("section"=w390, "value"=w381, "key"="FrameRate", "refnum"=w392) -> ("refnum out"=w391:T14)  [unwired: 1 in, 6 out]
            n249 = property on="Camera Settings" class="Clust (strict)"("Visible"=w393) -> ()  [unwired: 2 in, 2 out]
            n250 = local write "DB Camera Config"(w393) -> ()
            n251 = call-poly <vilib>:"Write Key.vi"("section"=w390, "value"=w380, "key"="Compression", "refnum"=w391) -> ("refnum out"=w377:T14)  [unwired: 1 in, 6 out]
            n252 = call <vilib>:"Close Config Data.vi"("refnum"=w377) -> ("file path"=w378:path)  [unwired: 2 in, 8 out]
            n253 = call <vilib>:"Open Config Data.vi"("configuration file path"=w378) -> ("refnum"=w376:T14)  [unwired: 8 in, 2 out]
          }
          frame True {
            n254 = property on="Camera Settings" class="Clust (strict)"("Visible"=TRUE) -> ()  [unwired: 2 in, 2 out]
          }
        }
      }
      event "Camera Settings": Value Change {
        n255 = event-data() -> ("NewVal"=w407:T2)  [unwired: 1 in]
        n256 = Index Array(array=w403) -> (element=w402:cluster{string[]})  [unwired: 1 in]
        n257 = Unbundle(w407) -> ("Frame Rate"=w398:i32, "Compression"=w397:i32, "Size"=w400:u16)
        n258 = Unbundle(w402) -> (w401:string[])
        n259 = Index Array(array=w401, index=w400) -> (element=w399:string)
        n260 = Format Into String(format string="%s   %dfps   %d%%", w399, w398, w397) -> (resulting string=w404:string)  [unwired: 2 in, 1 out]
        n261 = Build Array(w404) -> (w405:string[])
        n262 = property on="DB Camera Config" class="Bool (strict)"("Strings [4]"=w405) -> ()  [unwired: 2 in, 2 out]
      }
      event "Motor.Enable": Value Change {
        n263 = event-data() -> ("NewVal"=w413:bool)  [unwired: 1 in]
        n264 = Unbundle("Motor") -> ("Value"=w412:dbl)  [unwired: 1 out]
        n265 = Select(t=w412, s=w413, f=0.0) -> (s? t:f=w410:dbl)
        n266 = call <vilib>:"NT Write Number.vi"("Numeric"=w410, "Name"=w409) -> ()  [unwired: 9 in, 1 out]
      }
      event "Test Slider": Value Change {
        n267 = event-data() -> ("NewVal"=w416:dbl)  [unwired: 1 in]
        n268 = call <vilib>:"NT Write Number.vi"("Numeric"=w416, "Name"=w417) -> ()  [unwired: 9 in, 1 out]
      }
      event "On/Off": Value Change {
        n269 = event-data() -> ("NewVal"=w421:bool)  [unwired: 1 in]
        n270 = Boolean To (0,1)(Boolean=w421) -> (0, 1=w420:i16)
        n271 = call <vilib>:"NT Write Number.vi"("Numeric"=w420, "Name"=w419) -> ()  [unwired: 9 in, 1 out]
      }
      event "Rev/Fwd": Value Change {
        n272 = event-data() -> ("NewVal.Forward"=w429:bool, "NewVal.Reverse"=w428:bool)  [unwired: 1 in]
        n273 = Boolean To (0,1)(Boolean=w429) -> (0, 1=w425:i16)
        n274 = Boolean To (0,1)(Boolean=w428) -> (0, 1=w427:i16)
        n275 = Negate(x=w427) -> (-x=w426:i16)
        n276 = Add(x=w425, y=w426) -> (x+y=w424:i16)
        n277 = call <vilib>:"NT Write Number.vi"("Numeric"=w424, "Name"=w423) -> ()  [unwired: 9 in, 1 out]
      }
      event "Test Ring": Value Change {
        n278 = event-data() -> ("NewVal"=w433:u16)  [unwired: 1 in]
        n279 = property on="Test Ring" class="Ring (strict)"() -> ("Strings []"=w434:string[])  [unwired: 2 in, 2 out]
        n280 = Index Array(array=w434, index=w433) -> (element=w432:string)
        n281 = call <vilib>:"NT Write String.vi"("String"=w432, "Name"=w431) -> ()  [unwired: 9 in, 1 out]
      }
      event "Rec Mode": Value Change {
        # "Update globals for recording mode and path to read log from.\nClear when logging and let NetworkTables set path for vision to\nuse."
        n282 = event-data() -> ("NewVal"=w444:enum32{"Stop", "Record", "Playback"})  [unwired: 1 in]
        n283 = global write "WPI_DashboardLogging Global.vi" "Logging Filename"(path "") -> ()
        n284 = case shown="\"Stop\", \"Record\"" w444 {
          tunnel: w443 -> [_ w446 w454]
          tunnel: [_ _ w453] -> w440
          tunnel: [_ _ w452] -> _
          tunnel: w438 -> [_ _ w450]
          tunnel: cluster{i32, i32} {-250, 170} -> [_ _ w449]
          tunnel: [_ _ T16 {"Image Size"=TRUE, "Image Type"=TRUE, "Pixel Value"=TRUE, "ROI Information"=TRUE, "Zoom Factor"=FALSE} ("Image Information Shown:All Elements")] -> w436
          tunnel: [_ _ TRUE ("Zoom Factor")] -> w435
          frame Default {
          }
          frame "Stop", "Record" {
            # "Place Window too"
            n285 = invoke class="VI" method="FP.Close"(reference=w446) -> (reference out=w445:refnum<vi>)  [unwired: 2 in, 2 out]
            n286 = invoke class="VI" method="Abort VI"(reference=w445) -> ()  [unwired: 2 in, 3 out]
          }
          frame "Playback" {
            n287 = call "Open Playback Panel.vi"("Offset"=w449, "DB VI Ref"=w450, "Playback in"=w454) -> ("Playback out"=w451:refnum<vi>)  [unwired: 8 in]
            n288 = register-events(w451) -> (reference out=w453:refnum<event-registration>, error out=w452:errorcluster)  [unwired: 2 in]
          }
        }
        n289 = global write "WPI_DashboardLogging Global.vi" "Recording"(w444) -> ()
        n290 = property on="Camera Image" class="ImageControl"("Image Information Shown"=w436, "Image Information Visible"=w435) -> ()  [unwired: 2 in, 2 out]
        n291 = call <vilib>:"WPI_DashboardNT Log FieldName Cache.vi"("Operation"=enum16{"Lookup/Add", "Index", "Clear"}."Clear") -> ()  [unwired: 8 in, 3 out]
      }
      event Panel Close {
        w455 = enum32{"Stop", "Record", "Playback"}."Stop" ("Rec Mode")
        n292 = event-data() -> ()  [unwired: 1 in, 4 out]
        n293 = local write "Rec Mode"(w455) -> ()
        n294 = global write "WPI_DashboardLogging Global.vi" "Recording"(w455) -> ()
      }
      event Panel Close {
        # "Abort playback window and ourself"
        n295 = event-data() -> ()  [unwired: 1 in, 4 out]
        n296 = invoke class="VI" method="FP.Close"(reference=w460) -> (reference out=w459:refnum<vi>)  [unwired: 2 in, 2 out]
        n297 = invoke class="VI" method="Abort VI"(reference=w459) -> (error out=w458:errorcluster)  [unwired: 2 in, 2 out]
        n298 = invoke class="VI" method="Abort VI"(error in=w458) -> ()  [unwired: 2 in, 3 out]
      }
    }
  }
  n299 = Wait (ms)(milliseconds to wait=u32 500) -> ()  [unwired: 1 out]
  n300 = property on="On/Off" class="Bool (strict)"("Visible"=w31) -> ()  [unwired: 2 in, 2 out]
  n301 = property on="Motor" class="Clust (strict)"("Visible"=w31) -> ()  [unwired: 2 in, 2 out]
  n302 = property on="Progress" class="Clust (strict)"("Visible"=w31) -> ()  [unwired: 2 in, 2 out]
  n303 = property on="Test Ring" class="Ring (strict)"("Visible"=w31) -> ()  [unwired: 2 in, 2 out]
  n304 = property on="Rev/Fwd" class="Clust (strict)"("Visible"=w31) -> ()  [unwired: 2 in, 2 out]
  n305 = property on="Camera Settings" class="Clust (strict)"("Visible"=w31) -> ()  [unwired: 2 in, 2 out]
  n306 = local write "DB Camera Config"(w31) -> ()
  n307 = global write "WPI_DashboardLogging Global.vi" "Recording"(w14) -> ()
  n308 = local write "Rec Mode"(w14) -> ()
